vi "CreateStructures.vi"(7 "PythonConverter_BD in":refnum<class "PyConvBD.lvclass">, 8 "error in":errorcluster, 11 "Diagram in":refnum<class "Diagram.lvclass">) -> (0 "error out":errorcluster, 3 "Diagram out":refnum<class "Diagram.lvclass">, 4 "create structures":string, 5 "PythonConverter_BD out":refnum<class "PyConvBD.lvclass">)   [LabVIEW 2014, in "Diagram.lvclass"]
uses:
  Diagram.lvclass
  Python/PythonConverter_BD/PyConvBD.lvclass
  Python/Parsing/ClassTypeTD.ctl
  Diagram.lvclass/Diagram.ctl
  FlatSequence/FlatSequence.lvclass/FlatSequence.ctl
  FlatSequence/FlatSequence.lvclass
  Structure/Structure.lvclass
  FlatSequenceFrame/FlatSequenceFrame.lvclass
  Python/Parsing/Python Functions.lvlib
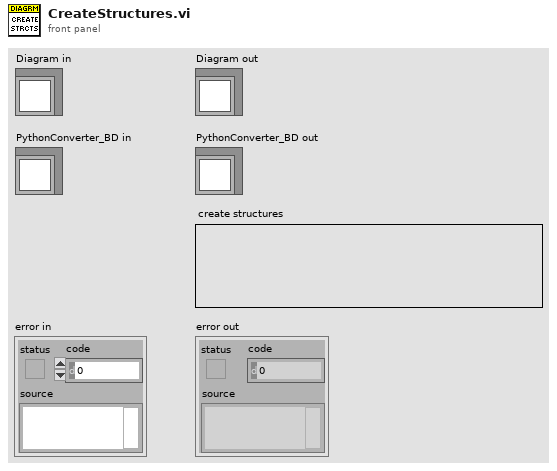
[diagram p1: front panel]
types:
  T1 = typedef "Python Functions.lvlib/ClassTypeTD.ctl" = enum16{"class", "function"}
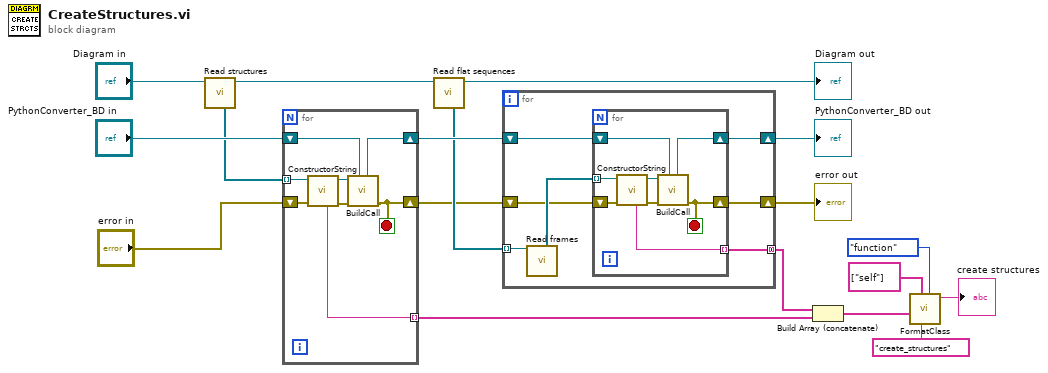
[diagram p0: block diagram]
diagram:
  n1 = call "Read structures.vi"("Diagram in"="Diagram in") -> ("Diagram out"=w1:refnum<class "Diagram.lvclass">, "structures"=w11:refnum<class "Structure.lvclass">[])  [unwired: 7 in]
  n2 = for {
    shift-right: [w22] -> w10
    shift-left: "PythonConverter_BD in" -> [w23]
    shift-right: [w21] -> w7
    shift-left: "error in" -> [w20]
    tunnel: [w26] -> w4 mode=indexing
    tunnel: w11 -> [w19] mode=indexing
    stop <- w21 stop-if-true
    n3 = call-dynamic "ConstructorString.vi"("error in"=w20, "Structure in"=w19) -> ("error out"=w25:errorcluster, "Structure out"=w24:refnum<class "Structure.lvclass">, "constructor"=w26:string)  [unwired: 5 in]
    n4 = call-dynamic "BuildCall.vi"("PythonConverter_BD in"=w23, "error in"=w25, "Structure in"=w24) -> ("error out"=w21:errorcluster, "PythonConverter_BD out"=w22:refnum<class "PyConvBD.lvclass">)  [unwired: 6 in, 1 out]
  }
  n5 = call "Read flat sequences.vi"("Diagram in"=w1) -> ("Diagram out"=→"Diagram out":refnum<class "Diagram.lvclass">, "flat sequences"=w8:refnum<class "FlatSequence.lvclass">[])  [unwired: 7 in]
  n6 = for {
    shift-right: [w32] -> w9
    shift-left: w10 -> [w33]
    tunnel: w8 -> [w31] mode=indexing
    shift-right: [w28] -> w6
    shift-left: w7 -> [w29]
    tunnel: [w27] -> w5 mode=concatenating
    n7 = call "Read frames.vi"("FlatSequence in"=w31) -> ("frames"=w30:refnum<class "FlatSequenceFrame.lvclass">[])  [unwired: 7 in, 1 out]
    n8 = for {
      shift-right: [w35] -> w32
      shift-left: w33 -> [w36]
      shift-right: [w34] -> w28
      shift-left: w29 -> [w40]
      tunnel: w30 -> [w41] mode=indexing
      tunnel: [w39] -> w27 mode=indexing
      stop <- w34 stop-if-true
      n9 = call-dynamic "ConstructorString.vi"("error in"=w40, "FlatSequenceFrame in"=w41) -> ("error out"=w37:errorcluster, "FlatSequenceFrame out"=w38:refnum<class "FlatSequenceFrame.lvclass">, "constructor"=w39:string)  [unwired: 5 in]
      n10 = call-dynamic "BuildCall.vi"("PythonConverter_BD in"=w36, "error in"=w37, "FlatSequenceFrame in"=w38) -> ("error out"=w34:errorcluster, "PythonConverter_BD out"=w35:refnum<class "PyConvBD.lvclass">)  [unwired: 6 in, 1 out]
    }
  }
  "error out" <- w6
  "PythonConverter_BD out" <- w9
  n11 = Build Array (concatenate)(w5, w4) -> (w3:string[])
  n12 = call "FormatClass.vi"("type"=ClassTypeTD."function", "name"="create_structures" ("initial string"), "parameters/ancestors"=string[] ["self"], "body"=w3) -> ("python"=→"create structures":string)  [unwired: 7 in]
